vi "start.vi"(8 "error in (no error)":errorcluster, 11 "NetworkPixelfly in":refnum<class "NetworkPixelfly.lvclass">) -> (0 "error out":errorcluster, 3 "NetworkPixelfly out":refnum<class "NetworkPixelfly.lvclass">)   [LabVIEW 2009, in "Hardware.lvlib" / "HWControllers.lvlib" / "NetworkPixelfly.lvclass"]
uses:
  NetworkPixelfly.lvclass
  Channels/Camera/PixelflySA/PixelflySA.lvclass
  NetworkCamera.lvclass
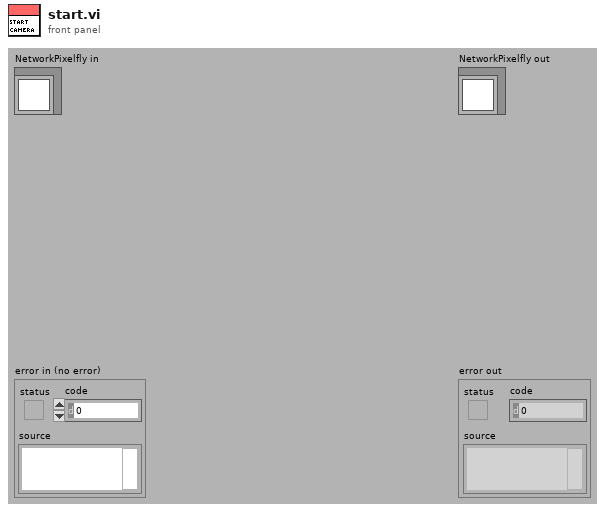
[diagram p1: front panel]
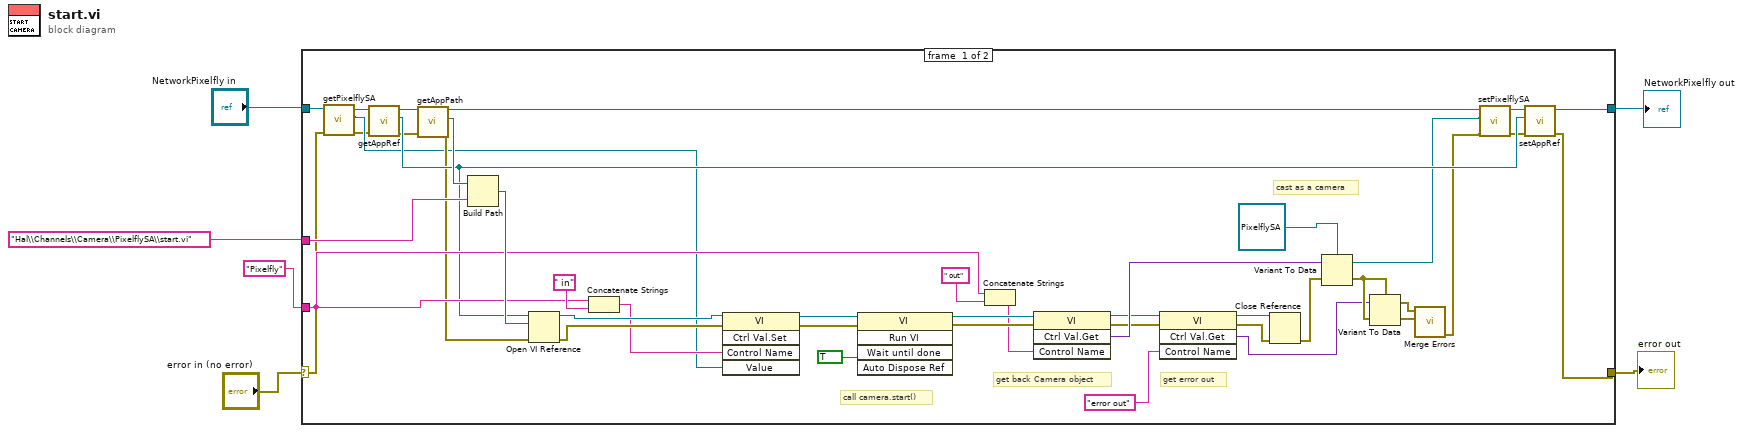
[diagram p0: block diagram]
diagram:
  n1 = case shown="No Error" "error in (no error)" {
    selector: "error in (no error)" -> [w13 w51]
    tunnel: [w28 w51] -> w2
    tunnel: [w30 w50] -> w1
    tunnel: "NetworkPixelfly in" -> [w14 w50]
    tunnel: "Hal\\Channels\\Camera\\PixelflySA\\start.vi" ("viPath") -> [w38 _]
    tunnel: "Pixelfly" ("Control name") -> [w35 _]
    frame #0 {
      # "get error out"
      # "get back Camera object"
      # "call camera.start()"
      # "cast as a camera"
      n2 = call "getPixelflySA.vi"("error in (no error)"=w13, "NetworkCamera in"=w14) -> ("error out"=w15:errorcluster, "PixelflySA.lvclass"=w16:refnum<class "PixelflySA.lvclass">, "NetworkCamera out"=w17:refnum<class "NetworkPixelfly.lvclass">)  [unwired: 7 in]
      n3 = call "getAppRef.vi"("error in (no error)"=w15, "NetworkCamera in"=w17) -> ("error out"=w19:errorcluster, "appRef"=w29:refnum<vi>, "NetworkCamera out"=w32:refnum<class "NetworkPixelfly.lvclass">)  [unwired: 7 in]
      n4 = call "getAppPath.vi"("error in (no error)"=w19, "NetworkCamera in"=w32) -> ("error out"=w18:errorcluster, "appPath"=w31:path, "NetworkCamera out"=w9:refnum<class "NetworkPixelfly.lvclass">)  [unwired: 7 in]
      n5 = Build Path(base path=w31, name or relative path=w38) -> (appended path=w49:path)
      n6 = Open VI Reference(application reference (local)=w29, vi path=w49, error in (no error)=w18) -> (vi reference=w40:refnum<vi>, error out=w39:errorcluster)  [unwired: 3 in]
      n7 = Concatenate Strings(w35, " in") -> (w36:string)
      n8 = invoke class="VI" method="Ctrl Val.Set"(reference=w40, error in=w39, "Control Name"=w36, "Value"=w16) -> (reference out=w48:refnum<vi>, error out=w47:errorcluster)  [unwired: 1 in, 3 out]
      n9 = invoke class="VI" method="Run VI"(reference=w48, error in=w47, "Wait until done"=TRUE) -> (reference out=w45:refnum<vi>, error out=w44:errorcluster)  [unwired: 2 in, 3 out]
      n10 = Concatenate Strings(w35, " out") -> (w33:string)
      n11 = invoke class="VI" method="Ctrl Val.Get"(reference=w45, error in=w44, "Control Name"=w33) -> (reference out=w42:refnum<vi>, error out=w26:errorcluster, "Get Control Value Variant"=w43:variant)  [unwired: 1 in, 1 out]
      n12 = invoke class="VI" method="Ctrl Val.Get"(reference=w42, error in=w26, "Control Name"="error out") -> (reference out=w27:refnum<vi>, error out=w25:errorcluster, "Get Control Value Variant"=w23:variant)  [unwired: 1 in, 1 out]
      n13 = Close Reference(reference=w27, error in (no error)=w25) -> (error out=w41:errorcluster)
      n14 = Variant To Data(error in=w41, Variant=w43, type=refnum<class "PixelflySA.lvclass"> refnum ("PixelflySA.lvclass")) -> (error out=w24:errorcluster, data=w8:refnum<class "PixelflySA.lvclass">)
      n15 = Variant To Data(error in=w24, Variant=w23, type=w24) -> (error out=w22:errorcluster, data=w21:errorcluster)
      n16 = call <vilib>:"Merge Errors.vi"("error in 2 (no error)"=w22, "error in 1 (no error)"=w21) -> ("error out"=w7:errorcluster)  [unwired: 5 in]
      n17 = call "setPixelflySA.vi"("error in (no error)"=w7, "PixelflySA.lvclass"=w8, "NetworkCamera in"=w9) -> ("error out"=w10:errorcluster, "NetworkCamera out"=w11:refnum<class "NetworkPixelfly.lvclass">)  [unwired: 7 in]
      n18 = call "setAppRef.vi"("error in (no error)"=w10, "appRef"=w29, "NetworkCamera in"=w11) -> ("error out"=w28:errorcluster, "NetworkCamera out"=w30:refnum<class "NetworkPixelfly.lvclass">)  [unwired: 7 in]
    }
    frame #1 {
    }
  }
  "error out" <- w2
  "NetworkPixelfly out" <- w1
